vi "DMLSFM_STROBE.vi"() -> ()   [LabVIEW 2017]
doc: "This example demonstrates how to generate a finite amount of digital data based off of a sample clock.\n\nSome hardware (e.g. M Series DAQ) must use an external sample clock for digital tasks. To view a complete list of available sample clock sources, consult the Device Routes table in Measurement and Automation Explorer.\n\nFor instructions on how to connect your signals to the DAQ device, refer to your device documentation."
uses:
  <vilib>/Utility/error.llb/DialogType.ctl
  <vilib>/DAQmx/write.llb/DAQmx Write (Analog 2D DBL NChan NSamp).vi
  <vilib>/DAQmx/create/channels.llb/DAQmx Create Channel (AO-Voltage-Basic).vi
  <vilib>/DAQmx/configure/timing.llb/DAQmx Timing (Sample Clock).vi
  <vilib>/DAQmx/configure/trigger.llb/DAQmx Start Trigger (Digital Edge).vi
  <vilib>/DAQmx/miscellaneous.llb/DAQmx Fill In Error Info.vi
  <resource>/objmgr/daqmx.rc
panel:
  out "error out":errorcluster
  in  "Start.Retriggerable":bool=TRUE
  in  "Digital Trigger Source":tag="/Dev4/PFI1"
  in  "Edge":i32(ring)=10280 items=["Rising"=10280, "Falling"=10171]
  in  "stop":bool
  in  "Sample Clock Source":tag="OnboardClock"
  out "Actual Sample Rate":dbl=1972.3865877712033 format="%0.2f"
  in  "Line(s)":tag="Dev4/ao0:1"
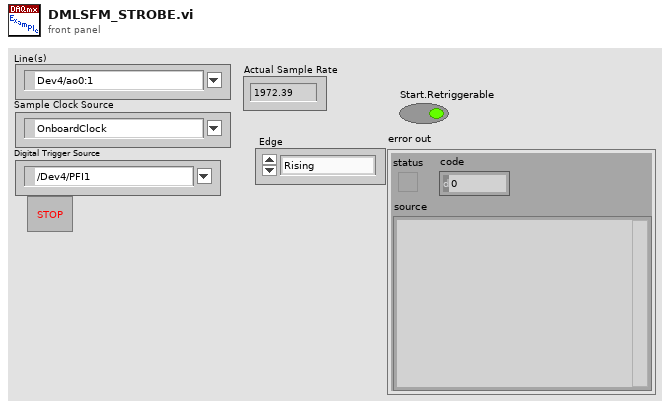
[diagram p1: front panel]
types:
  T1 = typedef "DialogType.ctl" = u16
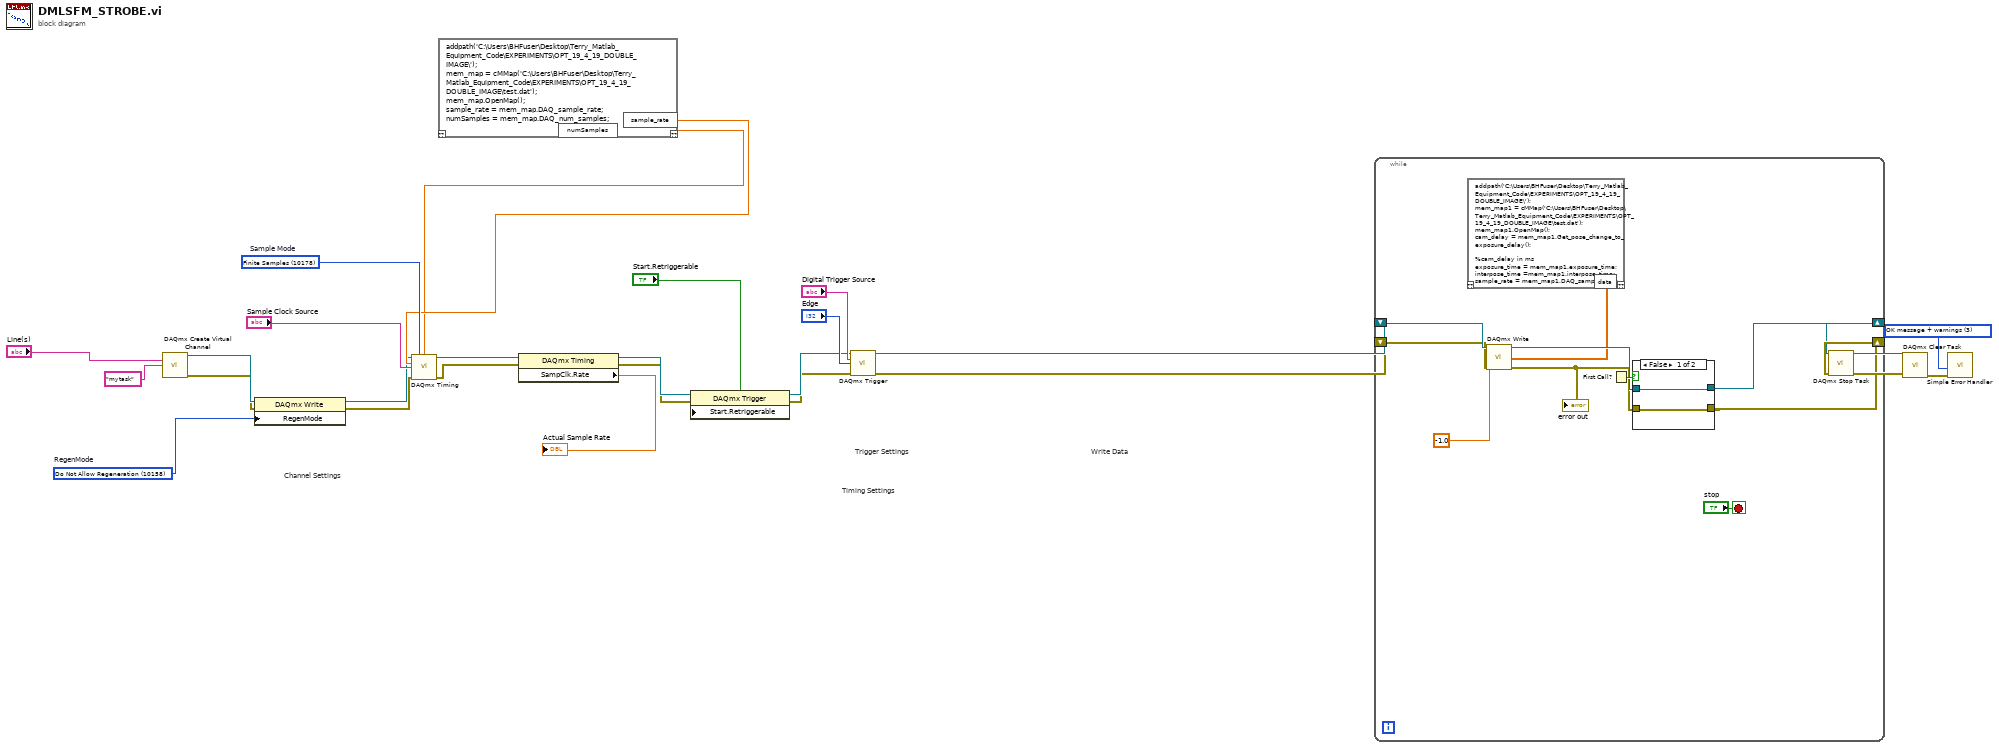
[diagram p0: block diagram]
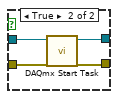
[diagram p2: hidden frame]
diagram:
  w4 = 10158 items=["Allow Regeneration"=10097, "Do Not Allow Regeneration"=10158]  # RegenMode
  w23 = T1 3 items=["no dialog", "OK message", "continue or stop message", "OK message + warnings", "continue/stop + warnings"] ("type of dialog (OK msg:1)")
  w24 = 10178 items=["Finite Samples"=10178, "Continuous Samples"=10123, "Hardware Timed Single Point"=12522]  # Sample Mode
  # "Trigger Settings"
  # "Timing Settings"
  # "Write Data"
  # "Channel Settings"
  n1 = call-poly <vilib>:"DAQmx Create Virtual Channel.vi"("physical channels"="Line(s)", "name to assign"="mytask") -> ("task out"=w8:refnum<k21>, "error out"=w6:errorcluster)  [unwired: 12 in]
  n2 = property class="DAQmx Write"(reference=w8, error in=w6, "RegenMode"=w4) -> (reference out=w7:refnum<k21>, error out=w5:errorcluster)
  n3 = script code="addpath('C:\\Users\\BHFuser\\Desktop\\Terry_Matlab_Equipment_Code\\EXPERIMENTS\\OPT_19_4_19_DOUBLE_IMAGE\\');\nmem_map = cMMap('C:\\Users\\BHFuser\\Desktop\\Terry_Matlab_Equipment_Code\\EXPERIMENTS\\OPT_19_4_19_DOUBLE_IMAGE\\test.dat');\nmem_map.OpenMap(); \nsample_rate = mem_map.DAQ_sample_rate;\nnumSamples = mem_map.DAQ_num_samples;"() -> ("sample_rate"=w19:dbl, "numSamples"=w18:dbl)  [unwired: 1 in, 1 out]
  n4 = call-poly <vilib>:"DAQmx Timing.vi"("task/channels in"=w7, "sample mode"=w24, "samples per channel"=w18, "rate"=w19, "source"="Sample Clock Source", "error in"=w5) -> ("task out"=w26:refnum<k21>, "error out"=w9:errorcluster)  [unwired: 8 in]
  n5 = property class="DAQmx Timing"(reference=w26, error in=w9) -> (reference out=w17:refnum<k21>, error out=w16:errorcluster, "SampClk.Rate"=→"Actual Sample Rate":dbl)
  n6 = property class="DAQmx Trigger"(reference=w17, error in=w16, "Start.Retriggerable"="Start.Retriggerable") -> (reference out=w15:refnum<k21>, error out=w14:errorcluster)
  n7 = call-poly <vilib>:"DAQmx Trigger.vi"("task/channels in"=w15, "source"="Digital Trigger Source", "edge"="Edge", "error in"=w14) -> ("task out"=w2:refnum<k21>, "error out"=w1:errorcluster)  [unwired: 10 in]
  n8 = while {
    shift-right: [w37] -> w10
    shift-left: w1 -> [w33]
    shift-right: [w36] -> w3
    shift-left: w2 -> [w35]
    stop <- "stop" stop-if-true
    n9 = script code="addpath('C:\\Users\\BHFuser\\Desktop\\Terry_Matlab_Equipment_Code\\EXPERIMENTS\\OPT_19_4_19_DOUBLE_IMAGE\\');\nmem_map1 = cMMap('C:\\Users\\BHFuser\\Desktop\\Terry_Matlab_Equipment_Code\\EXPERIMENTS\\OPT_19_4_19_DOUBLE_IMAGE\\test.dat');\nmem_map1.OpenMap(); \ncam_delay = mem_map1.Get_pose_change_to_exposure_delay();\n\n%cam_delay in ms\nexposure_time = mem_map1.exposure_time;\ninterpose_time =mem_map1.interpose_time;\nsample_rate = mem_map1.DAQ_sample_rate;\nsamples_per_pose = mem_map1.DAQ_samples_per_pose;\n\n\n\ndefocus = [50    40    30    20    10     0   -10   -20   -30   -40   -50   -30   -10    10    30];\nnumDefocus = numel(defocus);\nTTL_ON  = 5;\nTTL_OFF = 0;\n\n\nV_data = zeros(1, numDefocus*samples_per_pose);\ncam_data = zeros(1, numDefocus*samples_per_pose);\n\ncnt = 1;\nfor f = 1:numDefocus\n        for ff = 1 : samples_per_pose\n            fact = (ff - 1)/samples_per_pose;\n            V_data(cnt) = (1-fact)*defocus(f) + fact*defocus(mod(f,numDefocus)+1);\n            cnt = cnt + 1;\n        end\nend\n\n\nix_cam_start =  1 + cam_delay/1000 * sample_rate;\ncam_data( uint32(ix_cam_start) : uint32(ix_cam_start + exposure_time/1000*sample_rate)) = TTL_ON;\n\n        \n       \nnumSamples = numel(V_data);\nV_data = 0.271 - 0.00173 * V_data - 0.0000017*V_data.^2;\ndata = double([cam_data; V_data]);"() -> ("data"=w30:dbl[][])  [unwired: 1 in, 1 out]
    n10 = call-poly <vilib>:"DAQmx Write.vi"("task/channels in"=w35, "data"=w30, "timeout"=-1.0, "error in"=w33) -> ("task out"=w34:refnum<k21>, "error out"=w32:errorcluster)  [unwired: 9 in, 1 out]
    "error out" <- w32
    n11 = First Call?() -> (First Call?: T/F=w38:bool)
    n12 = case shown="False" w38 {
      tunnel: w34 -> [w40 w45]
      tunnel: w32 -> [w41 w44]
      tunnel: [w40 w43] -> w36
      tunnel: [w41 w42] -> w37
      frame False {
      }
      frame True {
        n13 = call <vilib>:"DAQmx Start Task.vi"("task/channels in"=w45, "error in"=w44) -> ("task out"=w43:refnum<k21>, "error out"=w42:errorcluster)  [unwired: 12 in]
      }
    }
  }
  n14 = call <vilib>:"DAQmx Stop Task.vi"("task/channels in"=w3, "error in"=w10) -> ("task out"=w12:refnum<k21>, "error out"=w11:errorcluster)  [unwired: 12 in]
  n15 = call <vilib>:"DAQmx Clear Task.vi"("task in"=w12, "error in"=w11) -> ("error out"=w29:errorcluster)  [unwired: 13 in]
  n16 = call <vilib>:"Simple Error Handler.vi"("type of dialog (OK msg:1)"=w23, "error in (no error)"=w29) -> ()  [unwired: 3 in, 5 out]
